vi "Read Joint Position.vi"(7 "Units (Encoder Counts)":T3=enum."Degrees", 8 "error in (no error)":errorcluster, 10 "Axis":T4=1 items=["Axis 1"=1, "Axis 2"=2, "Axis 3"=3, "Axis 4"=4, "Axis 5"=5, "Axis 6"=6, "Axis 7"=7, "Axis 8"=8], 11 "Board ID":T5=1 min=1 max=32 step=1) -> (0 "error out":errorcluster, 2 "Resource Output":T1=1 items=["Axis Control"=0, "Axis 1"=1, "Axis 2"=2, "Axis 3"=3, "Axis 4"=4, "Axis 5"=5, "Axis 6"=6, "Axis 7"=7, "Axis 8"=8, "Vector Space Control"=16, "Vector Space 1"=17, "Vector Space 2"=18, "Vector Space 3"=19, "Vector Space 4"=20, "Encoder Control"=32, "Encoder 1"=33, "Encoder 2"=34, "Encoder 3"=35, "Encoder 4"=36, "Encoder 5"=37, "Encoder 6"=38, "Encoder 7"=39, "Encoder 8"=40, "DAC Channel 1"=49, "DAC Channel 2"=50, "DAC Channel 3"=51, "DAC Channel 4"=52, "DAC Channel 5"=53, "DAC Channel 6"=54, "DAC Channel 7"=55, "DAC Channel 8"=56, "Stepper Output 1"=65, "Stepper Output 2"=66, "Stepper Output 3"=67, "Stepper Output 4"=68, "Stepper Output 5"=69, "Stepper Output 6"=70, "Stepper Output 7"=71, "Stepper Output 8"=72, "ADC Channel 1"=81, "ADC Channel 2"=82, "ADC Channel 3"=83, "ADC Channel 4"=84, "ADC Channel 5"=85, "ADC Channel 6"=86, "ADC Channel 7"=87, "ADC Channel 8"=88], 3 "Bd ID Out":T2, 5 "Joint Position":dbl)   [LabVIEW 2010]
doc: "Written for the PUMA 560. Reads the encoder position and corresponding joint angle of the given axis.\n\nOutput units can be specified as either degrees (default) or radians.\n\nNotes:\n\" Joint angles are computed using the formula: theta = (e/epr)*(2*pi/N)\nWhere theta is the joint angle, N is the gear ratio for the given axis (referenced from Peter Corke's paper titled \"The Unimation Puma Servo System\"), e is the current encoder count returned by the FlexMotion \"Read Position.flx\", 2*pi is 360 in the case of degrees units, and epr is the encoder counts per revolution of the axis."
uses:
  <vilib>/Motion/FlexMotion/CustomControls/CustomControls.llb/Axis To Read.flx
  Typedefs/Units_Enum.ctl
  <vilib>/Motion/FlexMotion/CustomControls/CustomControls.llb/Resource Out (Enum).flx
  Globals/AxisSpace.vi
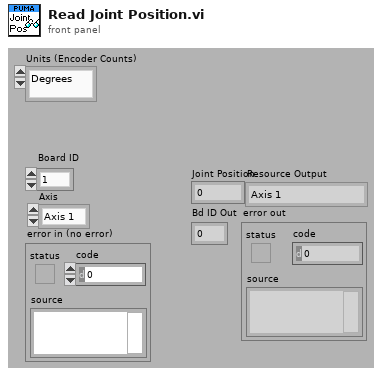
[diagram p1: front panel]
types:
  T1 = typedef "Resource Out (Enum).flx" = u16
  T2 = typedef "Bd Id Out" = u8
  T3 = typedef "Units_Enum.ctl" = enum16{"Radians", "Encoder Counts", "Revolutions", "Degrees"}
  T4 = typedef "Axis To Read.flx" = u16
  T5 = typedef "Board Id" = u8
  T6 = typedef "AxisSpaceCfg_ArrayofAxisCfg.ctl" = T7[]
  T7 = typedef "AxisCfg_cluster.ctl" = cluster{"Axis":T4, "Counts/Rev":dbl, "Gear Ratio":dbl, "Home Position":dbl}
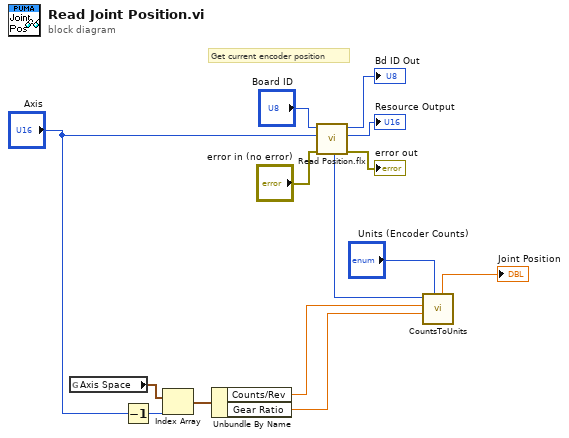
[diagram p0: block diagram]
diagram:
  # "Get current encoder position"
  n1 = global read "AxisSpace.vi" "Axis Space"() -> (w8:T6)
  n2 = Decrement(x="Axis") -> (x-1=w9:T4)
  n3 = Index Array(array=w8, index=w9) -> (element=w7:T7)
  n4 = Unbundle By Name(w7) -> ("Counts/Rev"=w2:dbl, "Gear Ratio"=w1:dbl)
  n5 = call <vilib>:"Read Position.flx"("error in (no error)"="error in (no error)", "Axis"="Axis", "Board ID"="Board ID") -> ("error out"=→"error out":errorcluster, "Resource Output"=→"Resource Output":T1, "Bd ID Out"=→"Bd ID Out":T2, "Position"=w3:i32)  [unwired: 3 in]
  n6 = call "CountsToUnits.vi"("Units (Encoder Counts)"="Units (Encoder Counts)", "Gear Ratio"=w1, "Counts/Rev"=w2, "Encoder Counts"=w3) -> ("Value in Units"=→"Joint Position":dbl)  [unwired: 7 in]
